vi "subvi_timer.vi"(8 "Timer Functions":T1=enum."Timed Out & Reset", 11 "Threshold Time (ms)":u32=100) -> (1 "Elapsed Time (ms)":u32, 3 "Timed Out?":bool=TRUE)   [LabVIEW 2014]
doc: "Timed Out: returns True when the Threshold Time (ms) is reached.\nTimed Out & Reset: returns True when the Threshold Time (ms) is reached and resets the Start Time so that the function will keep on timing out when reaching the threshold time.\nInitialise: initialises the Start Time. \nReset: resets the Start Time to zero."
uses:
  typedef_timer.ctl
panel:
  out "Threshold Time (ms)":u32
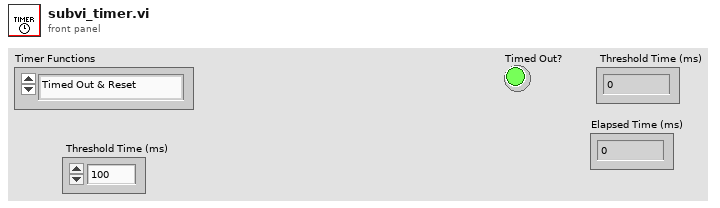
[diagram p1: front panel]
types:
  T1 = typedef "typedef_timer.ctl" = enum16{"Inside Time Window & Manual Reset", "Inside Time Window", "Reset", "Initialise", "Timed Out & Reset", "Timed Out"}
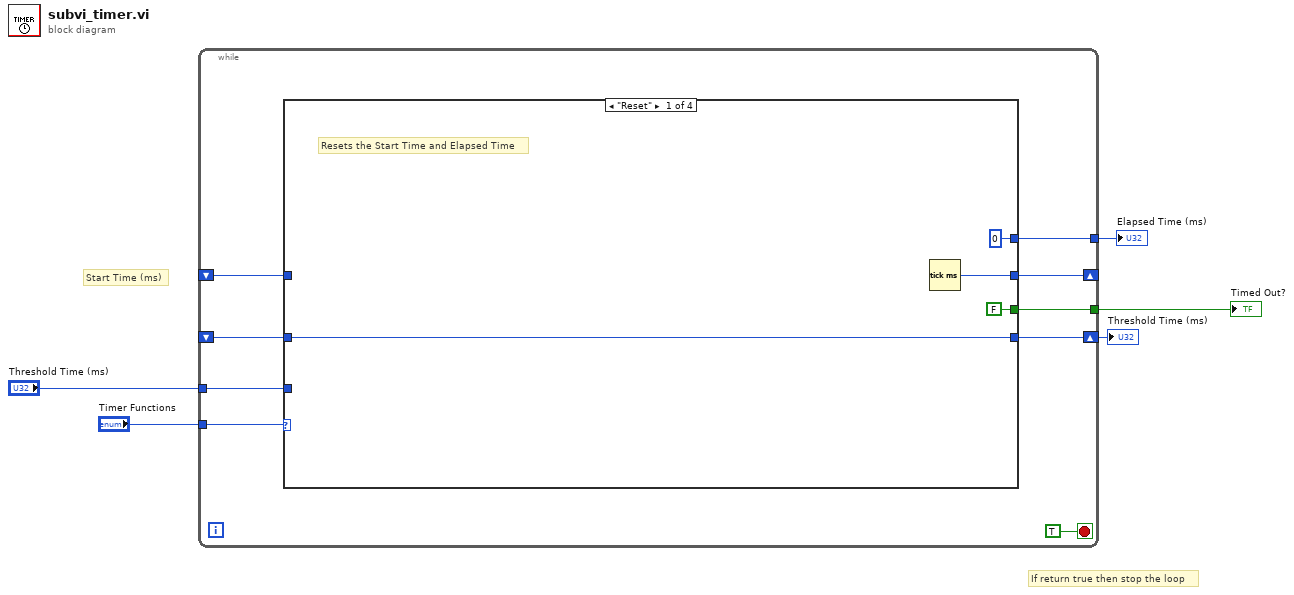
[diagram p0: block diagram]
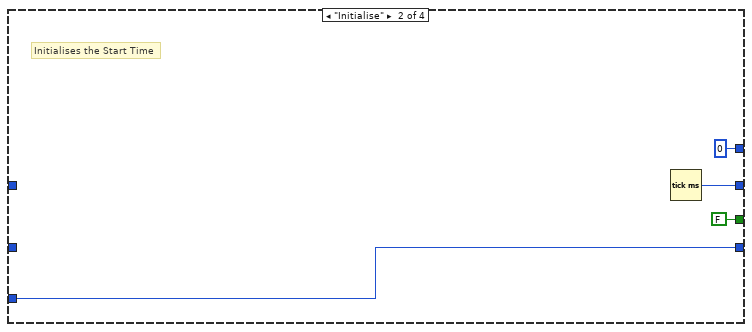
[diagram p2: hidden frame]
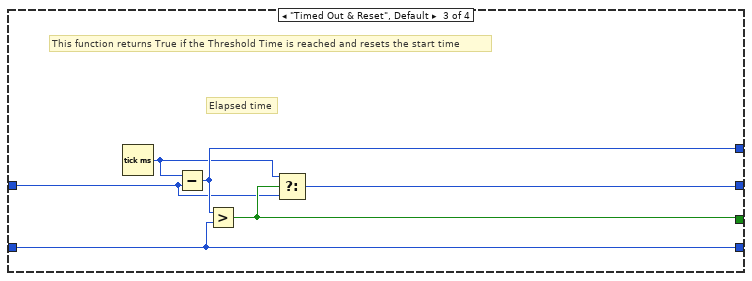
[diagram p3: hidden frame]
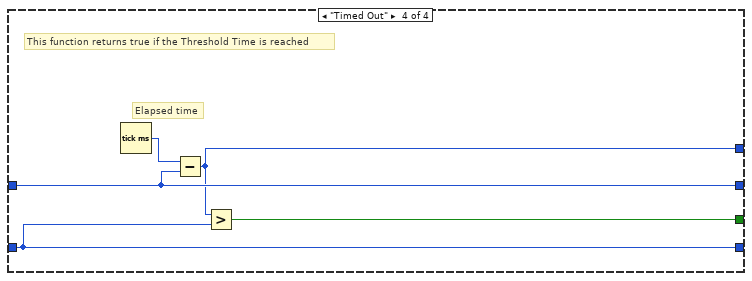
[diagram p4: hidden frame]
diagram:
  # "Start Time (ms)"
  # "If return true then stop the loop"
  n1 = while {
    tunnel: "Timer Functions" -> [w14]
    shift-right: [w11] -> _
    shift-left: _ -> [w13]
    shift-right: [w10] -> w2
    shift-left: _ -> [w12]
    tunnel: [w9] -> w4
    tunnel: "Threshold Time (ms)" -> [w7]
    tunnel: [w6] -> w1
    stop <- TRUE stop-if-true
    n2 = case shown="\"Reset\"" w14 {
      tunnel: w13 -> [_ _ w25 w32]
      tunnel: w12 -> [w16 _ w28 w31]
      tunnel: [w18 w20 w23 w32] -> w11
      tunnel: [w16 w22 w28 w31] -> w10
      tunnel: [FALSE FALSE w26 w30] -> w9
      tunnel: w7 -> [_ w22 _ _]
      tunnel: [u32 0 u32 0 w27 w29] -> w6
      frame "Reset" {
        # "Resets the Start Time and Elapsed Time"
        n3 = Tick Count (ms)() -> (millisecond timer value=w18:u32)
      }
      frame "Initialise" {
        # "Initialises the Start Time"
        n4 = Tick Count (ms)() -> (millisecond timer value=w20:u32)
      }
      frame "Timed Out & Reset", Default {
        # "Elapsed time"
        # "This function returns True if the Threshold Time is reached and resets the start time"
        n5 = Tick Count (ms)() -> (millisecond timer value=w24:u32)
        n6 = Subtract(x=w24, y=w25) -> (x-y=w27:u32)
        n7 = Greater?(x=w27, y=w28) -> (0:w26:bool)
        n8 = Select(t=w24, s=w26, f=w25) -> (s? t:f=w23:u32)
      }
      frame "Timed Out" {
        # "Elapsed time"
        # "This function returns true if the Threshold Time is reached"
        n9 = Tick Count (ms)() -> (millisecond timer value=w33:u32)
        n10 = Subtract(x=w33, y=w32) -> (x-y=w29:u32)
        n11 = Greater?(x=w29, y=w31) -> (0:w30:bool)
      }
    }
  }
  "Timed Out?" <- w4
  "Threshold Time (ms)" <- w2
  "Elapsed Time (ms)" <- w1
